vi "ConnectToServer.vi"(8 "error in (no error)":errorcluster, 11 "Client in":refnum<class "Client.lvclass">) -> (0 "error out":errorcluster, 3 "Client out":refnum<class "Client.lvclass">)   [LabVIEW 2021, in "Client.lvlib" / "Client.lvclass"]
uses:
  Client.lvclass
  C:/Program Files/National Instruments/LabVIEW 2021/vi.lib/ActorFramework/Actor/Actor.lvclass
  Client.lvclass/Client.ctl
  <vilib>/ActorFramework/Actor/Actor.lvclass/Actor.ctl
  <vilib>/ActorFramework/Message Enqueuer/Message Enqueuer.lvclass/Message Enqueuer.ctl
  <vilib>/NI/Actors/Network Endpoint Actors/Nested Endpoint/Nested Endpoint/Nested Endpoint.lvclass
  C:/Program Files/National Instruments/LabVIEW 2021/vi.lib/NI/Actors/Network Endpoint Actors/Network Endpoint/Network Endpoint/Network Endpoint.lvclass
  Client Messages/Connected Msg/Connected Msg.lvclass
  C:/Program Files/National Instruments/LabVIEW 2021/vi.lib/NI/Actors/Network Endpoint Actors/Nested Endpoint/Nested Endpoint Messages/Connected Msg/Connected Msg.lvclass
  <vilib>/NI/Actors/Network Endpoint Actors/Network Endpoint/Network Endpoint/Network Endpoint.lvclass/Network Endpoint.ctl
  <vilib>/NI/Actors/Network Endpoint Actors/Nested Endpoint/Nested Endpoint/Nested Endpoint.lvclass/Nested Endpoint.ctl
  <vilib>/ActorFramework/Message Enqueuer/Init from Existing Queue.vi
  <vilib>/ActorFramework/Message Enqueuer/Enqueue.vi
  <vilib>/ActorFramework/Stop Msg/Stop Msg.lvclass
  C:/Program Files/National Instruments/LabVIEW 2021/vi.lib/ActorFramework/Message/Message.lvclass
  <vilib>/NI/Actors/Network Endpoint Actors/Protocols/TCP Strategy/TCP Stream Initiator/TCP Stream Initiator.lvclass
  C:/Program Files/National Instruments/LabVIEW 2021/vi.lib/NI/Actors/Network Endpoint Actors/Abstract Classes/Message Stream/Message Stream.lvclass
  <vilib>/ActorFramework/Message Priority Queue/Priority Enqueue.vi
  <vilib>/ActorFramework/Message Enqueuer/Message Enqueuer.lvclass
  <vilib>/ActorFramework/Actor/Actor.lvclass
  <vilib>/NI/Actors/Network Endpoint Actors/Network Endpoint/Network Endpoint/Network Endpoint.lvclass
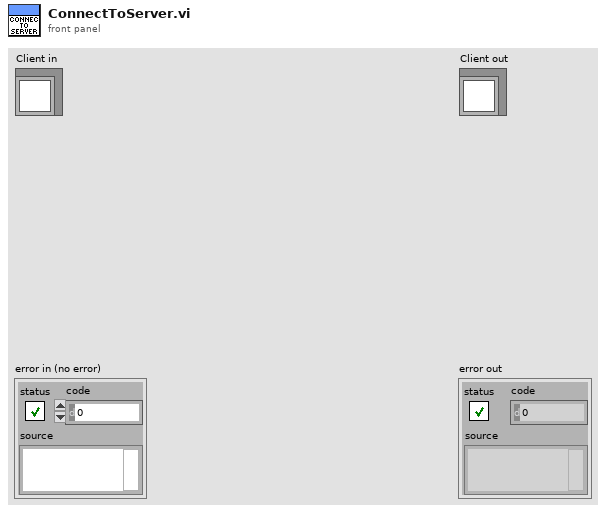
[diagram p1: front panel]
types:
  T1 = enum8{"Enabled", "Disabled", "Disabled and Grayed Out"}
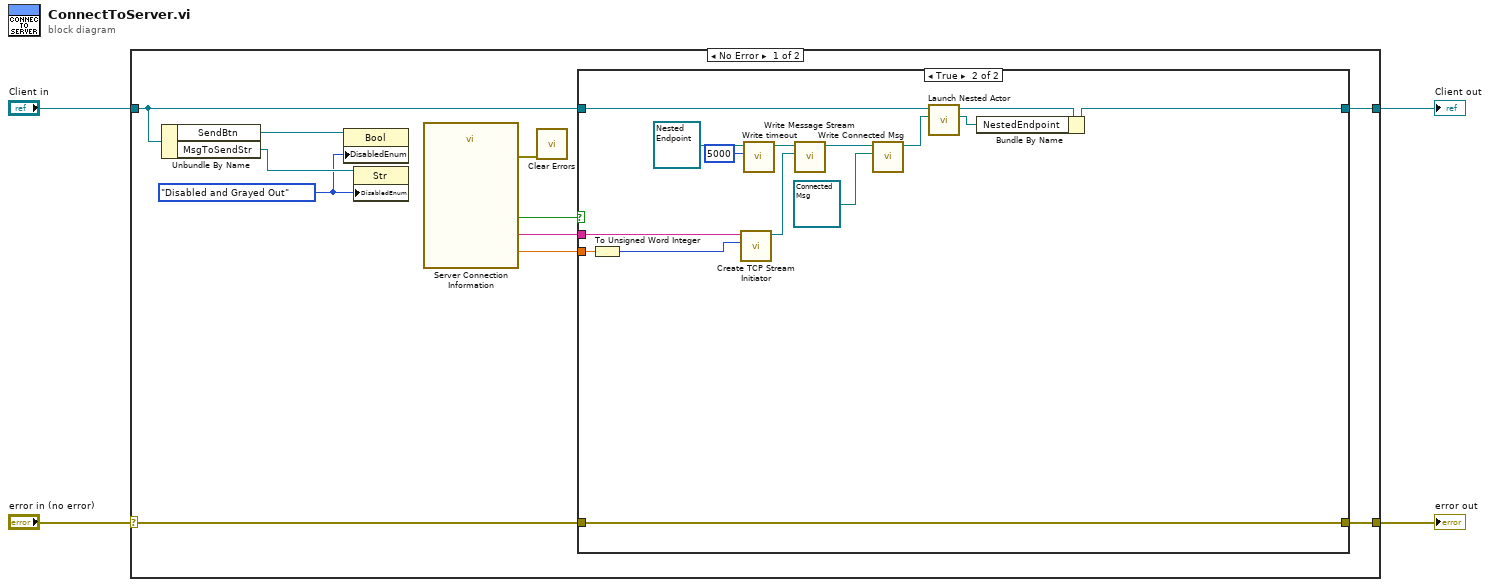
[diagram p0: block diagram]
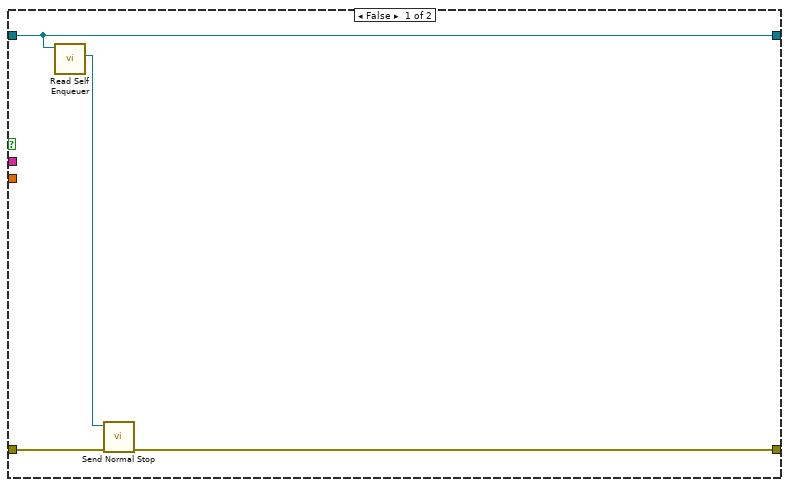
[diagram p2: hidden frame]
diagram:
  n1 = case shown="No Error" "error in (no error)" {
    selector: "error in (no error)" -> [w10 w36]
    tunnel: [w11 w36] -> w3
    tunnel: [w9 w35] -> w1
    tunnel: "Client in" -> [w8 w35]
    frame No Error {
      w5 = T1."Disabled and Grayed Out" ("Disabled")
      n2 = Unbundle By Name(w8) -> ("SendBtn"=w7:refnum<vi>, "MsgToSendStr"=w6:refnum<vi>)
      n3 = property class="Bool"(reference=w7, "DisabledEnum"=w5) -> ()  [unwired: 1 in, 2 out]
      n4 = property class="Str"(reference=w6, "DisabledEnum"=w5) -> ()  [unwired: 1 in, 2 out]
      n5 = call "Server Connection Information"() -> ("Port"=w12:dbl, "IP Address"=w13:string, "OK"=w15:bool, "error out"=w14:errorcluster)  [unwired: 16 in]
      n6 = call <vilib>:"Clear Errors.vi"("error in (no error)"=w14) -> ()  [unwired: 5 in, 2 out]
      n7 = case shown="True" w15 {
        tunnel: w13 -> [_ w27]
        tunnel: w12 -> [_ w26]
        tunnel: [w18 w34] -> w11
        tunnel: w10 -> [w19 w34]
        tunnel: w8 -> [w17 w33]
        tunnel: [w17 w23] -> w9
        frame False {
          n8 = call <vilib>:"Read Self Enqueuer.vi"("Actor"=w17) -> ("Self Enqueuer"=w16:refnum<class "Message Enqueuer.lvclass">)  [unwired: 10 in]
          n9 = call <vilib>:"Send Normal Stop.vi"("error in (no error)"=w19, "Message Enqueuer"=w16) -> ("error out"=w18:errorcluster)  [unwired: 9 in]
        }
        frame True {
          n10 = To Unsigned Word Integer(number=w26) -> (unsigned 16bit integer=w25:u16)
          n11 = call <vilib>:"Create TCP Stream Initiator.vi"("Remote Port"=w25, "Remote Address"=w27) -> ("TCP Stream Initiator"=w28:refnum<class "TCP Stream Initiator.lvclass">)  [unwired: 9 in]
          n12 = call <vilib>:"Write timeout.vi"("timeout"=5000, "Network Endpoint in"=refnum<class "Nested Endpoint.lvclass"> refnum ("Nested Endpoint.lvlib:Nested Endpoint.lvclass")) -> ("Network Endpoint out"=w29:refnum<class "Nested Endpoint.lvclass">)  [unwired: 9 in]
          n13 = call <vilib>:"Write Message Stream.vi"("Message Stream"=w28, "Network Endpoint in"=w29) -> ("Network Endpoint out"=w24:refnum<class "Nested Endpoint.lvclass">)  [unwired: 9 in]
          n14 = call <vilib>:"Write Connected Msg.vi"("Nested Endpoint.lvlib:Connected Msg.lvclass"=refnum<class "Connected Msg.lvclass"> refnum ("Client.lvlib:Connected Msg.lvclass"), "Nested Endpoint in"=w24) -> ("Nested Endpoint out"=w21:refnum<class "Nested Endpoint.lvclass">)  [unwired: 9 in]
          n15 = call <vilib>:"Launch Nested Actor.vi"("Nested Actor"=w21, "Caller Actor in"=w33) -> ("Nested Actor's Enqueuer"=w22:refnum<class "Message Enqueuer.lvclass">, "Caller Actor out"=w32:refnum<class "Client.lvclass">)  [unwired: 7 in, 1 out]
          n16 = Bundle By Name(cluster=w32, "NestedEndpoint"=w22) -> (w23:refnum<class "Client.lvclass">)
        }
      }
    }
    frame Error {
    }
  }
  "error out" <- w3
  "Client out" <- w1
